vi "JJMCclase8.vi"() -> ()   [LabVIEW 2013]
panel:
  out "Velocidad Minima":dbl
  out "Velocidad Maxima":dbl
  in  "encender":bool
  out "rango 151-220":bool
  out "rango 101-150":bool
  out "rango1-100":bool
  out "151-220":dbl
  out "101-150":dbl
  out "1-100":dbl
  out "Gauge":dbl(knob) scale=0.0..220.0
  # "se tiene que contar cuantas veces la velocidad se genera en cada una de los rangos y se enciende el led que corresponde a\ncada uno de los rangos.\nhacerlo hasta apagar el auto"
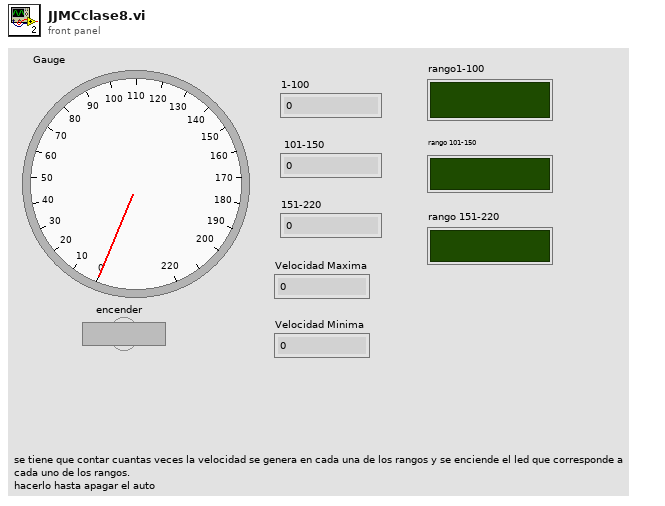
[diagram p1: front panel]
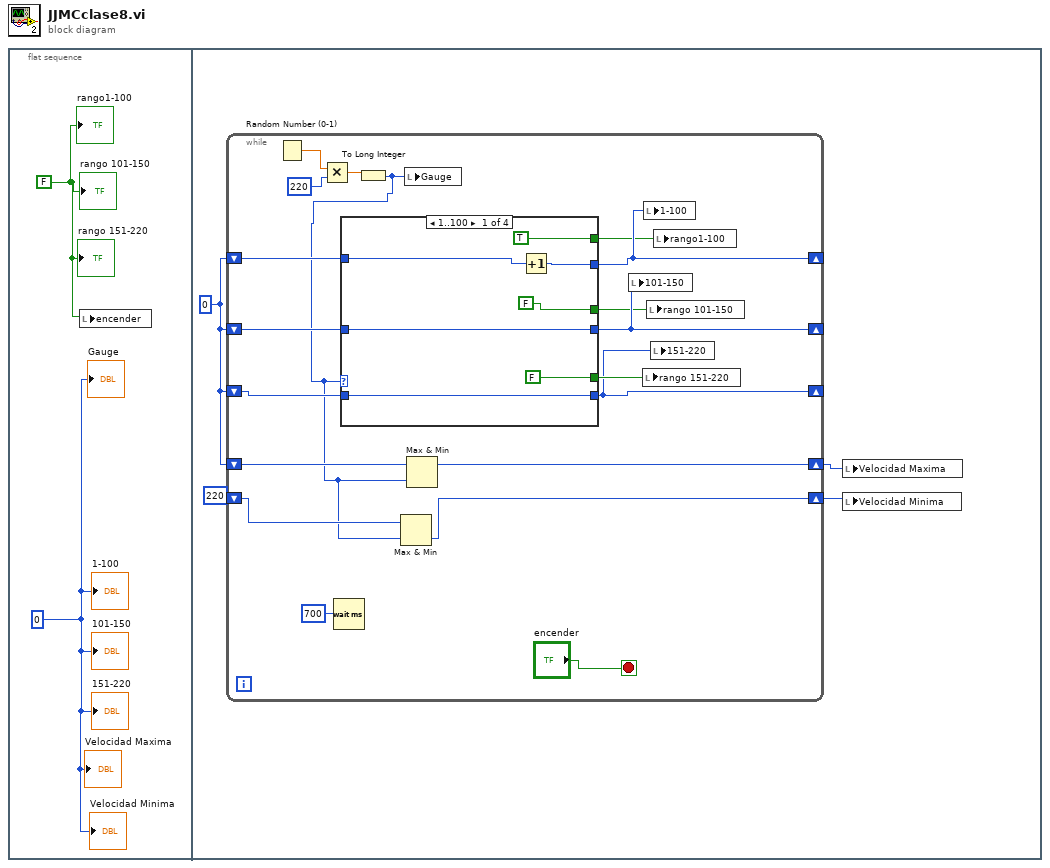
[diagram p0: block diagram]
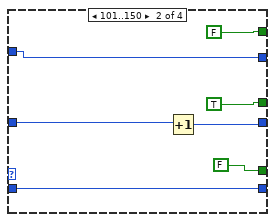
[diagram p2: hidden frame]
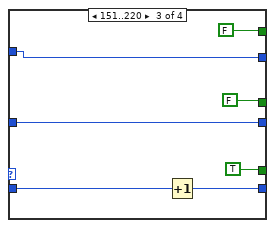
[diagram p3: hidden frame]
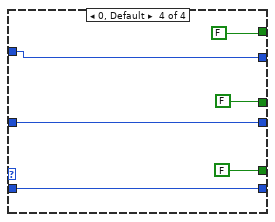
[diagram p4: hidden frame]
diagram:
  n1 = flat-sequence {
    frame #0 {
      w1 = 0
      w2 = FALSE
      n2 = local write "encender"(w2) -> ()
      "Gauge" <- w1
      "1-100" <- w1
      "101-150" <- w1
      "151-220" <- w1
      "rango1-100" <- w2
      "rango 101-150" <- w2
      "rango 151-220" <- w2
      "Velocidad Maxima" <- w1
      "Velocidad Minima" <- w1
    }
    frame #1 {
      w6 = 0
      n3 = while {
        shift-right: [w18] -> _
        shift-left: w6 -> [w21]
        shift-right: [w16] -> _
        shift-left: w6 -> [w20]
        shift-right: [w13] -> _
        shift-left: w6 -> [w19]
        shift-right: [w10] -> w4
        shift-left: w6 -> [w11]
        shift-right: [w9] -> w3
        shift-left: 220 -> [w8]
        stop <- "encender" stop-if-true
        n4 = Random Number (0-1)() -> (number: 0 to 1=w23:dbl)
        n5 = Multiply(x=w23, y=220) -> (x*y=w22:dbl)
        n6 = Wait (ms)(milliseconds to wait=700) -> ()  [unwired: 1 out]
        n7 = To Long Integer(number=w22) -> (32bit integer=w7:i32)
        n8 = case shown="1..100" w7 {
          tunnel: [w29 w39 w45 w52] -> w18
          tunnel: w21 -> [w30 w39 w45 w52]
          tunnel: [w32 w37 w44 w51] -> w16
          tunnel: w20 -> [w32 w38 w44 w51]
          tunnel: [w31 w36 w41 w50] -> w13
          tunnel: w19 -> [w31 w36 w40 w50]
          tunnel: [TRUE FALSE FALSE FALSE] -> w17
          tunnel: [FALSE TRUE FALSE FALSE] -> w15
          tunnel: [FALSE FALSE TRUE FALSE] -> w14
          frame 1..100 {
            n9 = Increment(x=w30) -> (x+1=w29:i32)
          }
          frame 101..150 {
            n10 = Increment(x=w38) -> (x+1=w37:i32)
          }
          frame 151..220 {
            n11 = Increment(x=w40) -> (x+1=w41:i32)
          }
          frame 0, Default {
          }
        }
        n12 = Max & Min(x=w8, y=w7) -> (min(x,y)=w9:i32)  [unwired: 1 out]
        n13 = local write "Gauge"(w7) -> ()
        n14 = Max & Min(x=w11, y=w7) -> (max(x,y)=w10:i32)  [unwired: 1 out]
        n15 = local write "101-150"(w16) -> ()
        n16 = local write "rango 151-220"(w14) -> ()
        n17 = local write "1-100"(w18) -> ()
        n18 = local write "rango 101-150"(w15) -> ()
        n19 = local write "151-220"(w13) -> ()
        n20 = local write "rango1-100"(w17) -> ()
      }
      n21 = local write "Velocidad Maxima"(w4) -> ()
      n22 = local write "Velocidad Minima"(w3) -> ()
    }
  }
